vi "OpenAllNodes.vi"   [LabVIEW 2012]
doc: "Opens all running nodes"
uses:
  <userlib>/ROSforLV/ROS/Code/SubVIs/_ROSControl.ctl
  <userlib>/ROSforLV/ROS/Code/SubVIs/_ROSDirection.ctl
  <userlib>/ROSforLV/ROS/Code/_ROSDefinition.vi
types:
  T1 = typedef "_ROSControl.ctl" = cluster{"topic port":u16, "Node":string, "topic":string, "type":string, "node port":u16, "error ":errorcluster, "Direction":T2, "Update (ms)":u16, "queue size":u16}
  T2 = typedef "_ROSDirection.ctl" = enum16{"Node", "Publisher", "Subscriber", "Service Client"}
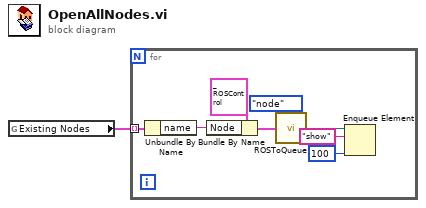
[diagram p0: block diagram]
diagram:
  n1 = global read "_ROSDefinition.vi" "Existing Nodes"() -> (w1:cluster{"name":string, "Port":u16}[])
  n2 = for {
    tunnel: w1 -> [w4] mode=indexing
    n3 = Unbundle By Name(w4) -> ("name"=w3:string)
    n4 = Bundle By Name(cluster=T1 {"topic port"=0, "Node"="/fred", "topic"="/robot/head/command_head_nod", "type"="std_msgs/Bool", "node port"=59377, "error "={"status"=FALSE, "code"=0, "source"=""}, "Direction"=enum."Publisher", "Update (ms)"=1, "queue size"=1} ("ROS"), "Node"=w3) -> (w6:T1)
    n5 = call <userlib>:"ROSToQueue.vi"("ROS"=w6, "Name"=enum16{"topic", "node"}."node") -> ("queue"=w8:refnum<queue>)  [unwired: 2 in, 1 out]
    n6 = Enqueue Element(queue=w8, element="show", timeout in ms (-1)=100) -> ()  [unwired: 1 in, 3 out]
  }
